vi "SetGetClass.vi"(7 "Set (f)":bool, 11 "Class In":refnum<class "SensorBase.lvclass">) -> (3 "Class Out":refnum<class "SensorBase.lvclass">)   [LabVIEW 2018, in "SensorPlugins.lvlib"]
uses:
  SensorBaseClass/SensorBase.lvclass
  SensorPlugins.lvlib
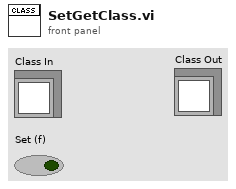
[diagram p1: front panel]
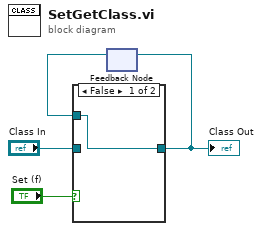
[diagram p0: block diagram]
diagram:
  n1 = feedback #1() -> (w1:refnum<class "SensorBase.lvclass">)  [unwired: 1 in]
  n2 = case shown="False" "Set (f)" {
    tunnel: [w5 w6] -> w3
    tunnel: "Class In" -> [_ w6]
    tunnel: w1 -> [w5 _]
    frame False {
    }
    frame True {
    }
  }
  "Class Out" <- w3
  n3 = feedback-in #1(w3) -> ()
